vi "getPath.vi"(8 "error in TCP":errorcluster, 11 "connection ID in":refnum<k5>) -> (0 "error out TCP":errorcluster, 2 "name vi":string, 3 "connection ID out":refnum<k5>)   [LabVIEW 2010]
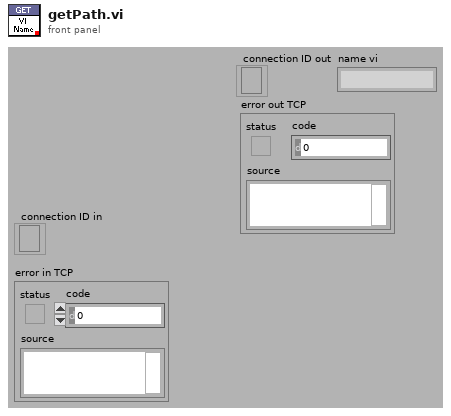
[diagram p1: front panel]
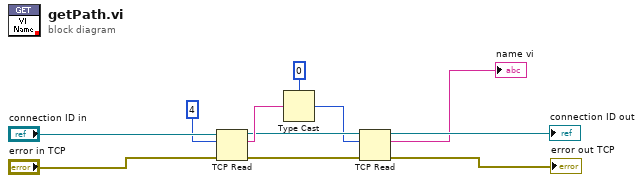
[diagram p0: block diagram]
diagram:
  n1 = TCP Read(connection ID="connection ID in", bytes to read=4, error in (no error)="error in TCP") -> (connection ID out=w6:refnum<k5>, data out=w8:string, error out=w5:errorcluster)  [unwired: 2 out]
  n2 = Type Cast(type=0, x=w8) -> (*(type *) &x=w4:i32)
  n3 = TCP Read(connection ID=w6, bytes to read=w4, error in (no error)=w5) -> (connection ID out=→"connection ID out":refnum<k5>, data out=→"name vi":string, error out=→"error out TCP":errorcluster)  [unwired: 2 out]
